vi "NI-DCPower Source DC Voltage.vi"(0 "Vin SMU":refnum<k15>="Dev1", 1 "Current Limit":dbl=0.01 format="%.3p", 2 "Current Limit Range":dbl=0.01 format="%.3p", 5 "Vin SMU Channel":string="0", 7 "Voltage Level":dbl=2.0 format="%.5p", 9 "Voltage Level Range":dbl=6.0 format="%.5p", 11 "error in":errorcluster) -> (4 "Voltage Measurement":dbl, 6 "Current Measurement":dbl, 15 "error out":errorcluster)   [LabVIEW 2020, in "SMU.lvlib"]
doc: "Demonstrates how to use the DC Voltage Output Function to force an output voltage. This example initializes a session, configures the Output Function, Sense, Autorange, Voltage Level and Current Limit, initiates generation, waits for a specified delay, and measures the voltage and current output. This example uses Single Point source mode."
uses:
  SMU.lvlib
  controls/Configuration.ctl
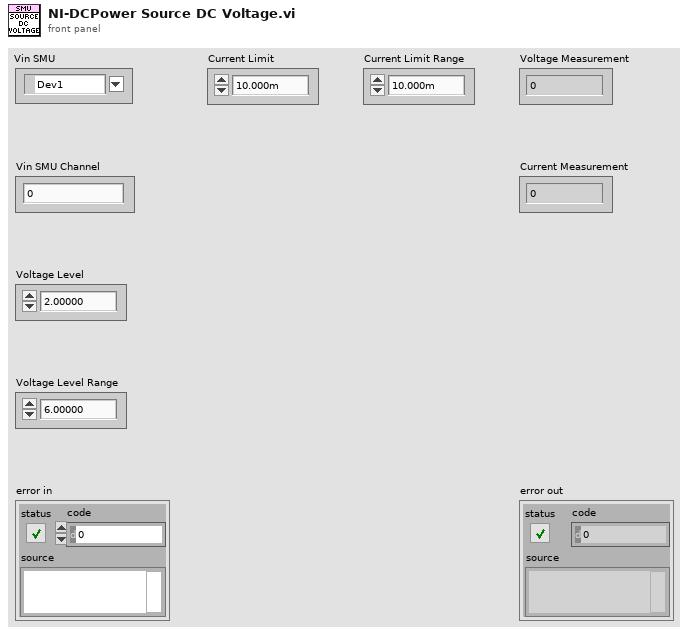
[diagram p1: front panel]
types:
  T1 = typedef "SMU.lvlib/Configuration.ctl" = cluster{"Voltage Level":dbl, "Voltage Level Range":dbl, "Current Limit":dbl, "Current Limit Range":dbl}
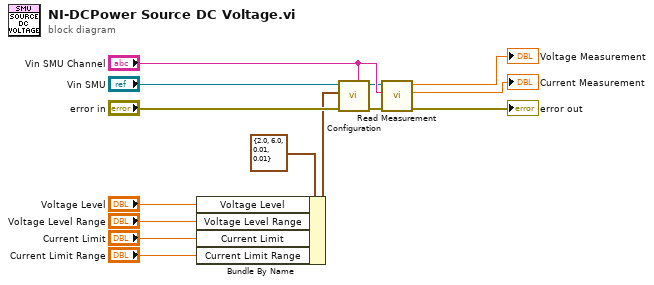
[diagram p0: block diagram]
diagram:
  n1 = Bundle By Name(cluster=T1 {"Voltage Level"=2.0, "Voltage Level Range"=6.0, "Current Limit"=0.01, "Current Limit Range"=0.01} ("Cluster"), "Voltage Level"="Voltage Level", "Voltage Level Range"="Voltage Level Range", "Current Limit"="Current Limit", "Current Limit Range"="Current Limit Range") -> (w1:T1)
  n2 = call "Configuration.vi"("Vin SMU Channel"="Vin SMU Channel", "error in (no error)"="error in", "Config"=w1, "IVI Refnum in"="Vin SMU") -> ("error out"=w3:errorcluster, "IVI Refnum out"=w4:refnum<k15>)  [unwired: 6 in]
  n3 = call "Read Measurement.vi"("error in (no error)"=w3, "Vin SMU Channel"="Vin SMU Channel", "IVI Refnum in"=w4) -> ("error out"=→"error out":errorcluster, "Current"=→"Current Measurement":dbl, "Voltage"=→"Voltage Measurement":dbl)  [unwired: 6 in]
